vi "Recall AP Sx State.vi"(8 "error in (no error)":errorcluster caption="错误输入（无错误）", 10 "asicName":string, 11 "asicHandle":i32) -> (0 "error out":errorcluster caption="错误输出", 2 "asicName out":string, 3 "function return":i32)   [LabVIEW 2018]
doc: "extern int __stdcall RecallAPSxState (int asicHandle, IN char * asicName);"
uses:
  APSx.dll/APSx.dll
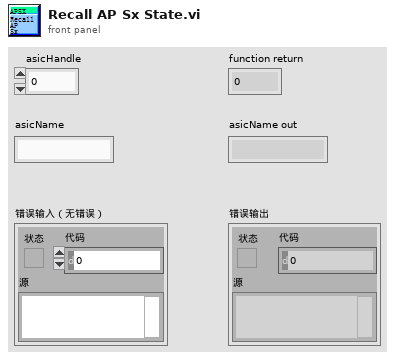
[diagram p1: front panel]
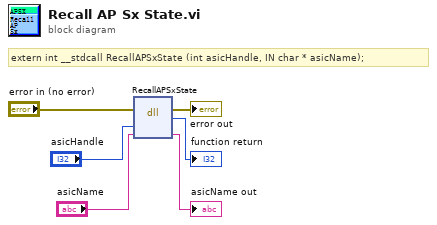
[diagram p0: block diagram]
diagram:
  # "extern int __stdcall RecallAPSxState (int asicHandle, IN char * asicName);"
  n1 = dll-call lib="PTH2[abs D项目Feng恒隆项目Labview传感器对中台SourcesAPSx.dllAPSx.*" fn="RecallAPSxState"(error in="error in (no error)", "asicHandle"="asicHandle", "asicName"="asicName") -> (error out=→"error out":errorcluster, →"function return":i32, "asicName"=→"asicName out":string)  [unwired: 3 in, 1 out]
